vi "readMatFile.vi"(7 "Path":path, 8 "error in (no error)":errorcluster, 9 "Skip Col Idx":i32[](array[numeric]), 10 "Skip Row Idx":i32[](array[numeric]), 11 "MatOper in":refnum<class "MatOper.lvclass">) -> (0 "error out":errorcluster, 2 "Matrix":dbl[][](array[numeric]), 3 "MatOper out":refnum<class "MatOper.lvclass">)   [LabVIEW 2016, in "MatOper.lvclass"]
doc: "Read the 2D matrix data from file."
uses:
  MatOper.lvclass
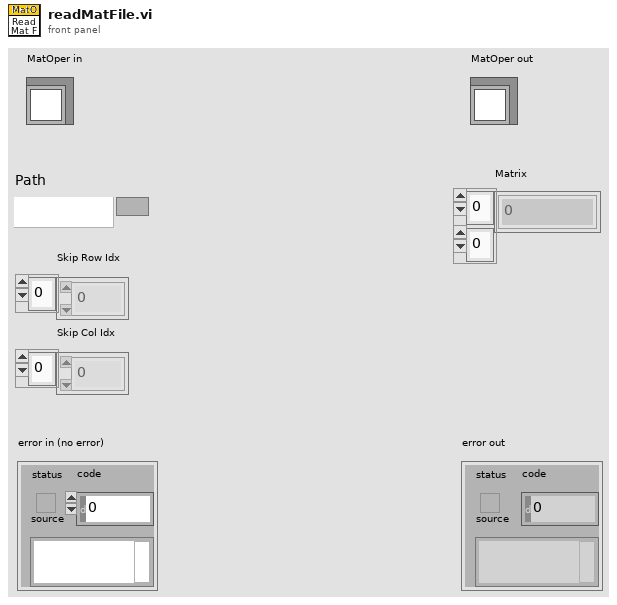
[diagram p1: front panel]
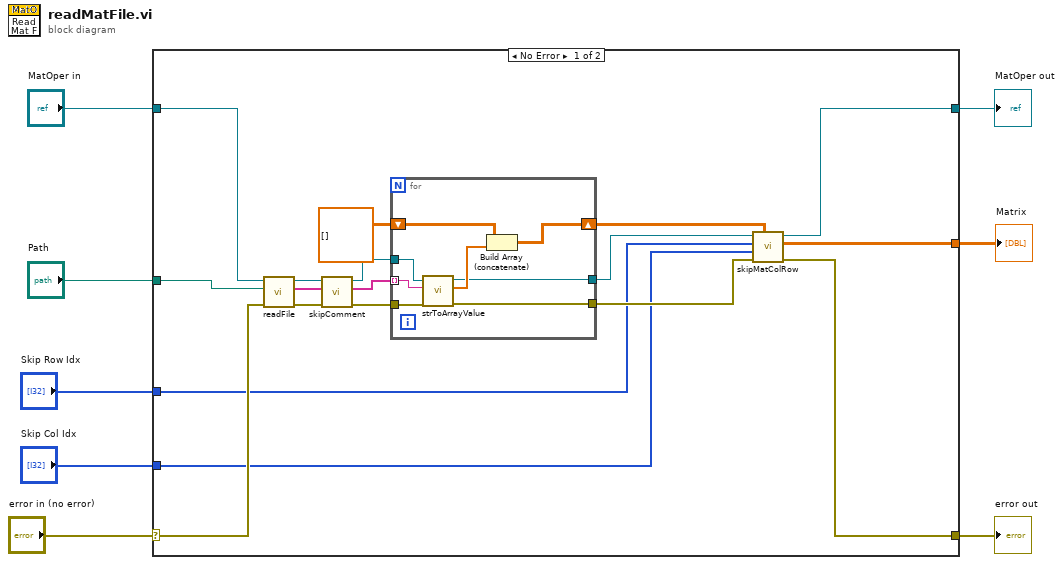
[diagram p0: block diagram]
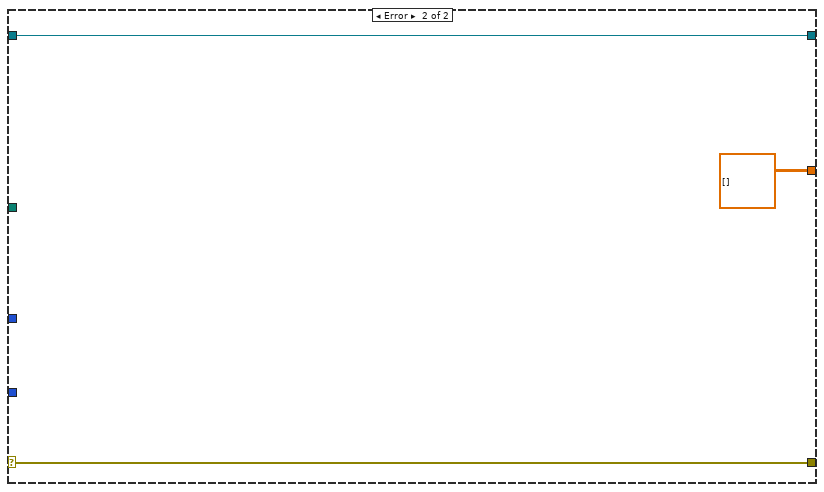
[diagram p2: hidden frame]
diagram:
  n1 = case shown="No Error" "error in (no error)" {
    selector: "error in (no error)" -> [w20 w37]
    tunnel: [w21 w37] -> w7
    tunnel: [w9 w36] -> w5
    tunnel: "MatOper in" -> [w10 w36]
    tunnel: [w22 dbl[][] [] ("Sub-Array")] -> w4
    tunnel: "Path" -> [w19 _]
    tunnel: "Skip Row Idx" -> [w18 _]
    tunnel: "Skip Col Idx" -> [w17 _]
    frame No Error {
      n2 = call "readFile.vi"("error in (no error)"=w20, "Path"=w19, "MatOper in"=w10) -> ("error out"=w15:errorcluster, "Array"=w26:string[], "MatOper out"=w13:refnum<class "MatOper.lvclass">)  [unwired: 6 in]
      n3 = call "skipComment.vi"("error in (no error)"=w15, "Content"=w26, "MatOper in"=w13) -> ("error out"=w14:errorcluster, "Modified Content"=w25:string[], "MatOper out"=w12:refnum<class "MatOper.lvclass">)  [unwired: 6 in]
      n4 = for {
        tunnel: w25 -> [w29] mode=indexing
        shift-right: [w32] -> w16
        shift-left: dbl[][] [] -> [w33]
        tunnel: w14 -> [w31]
        tunnel: [w30] -> w23
        tunnel: w12 -> [w28]
        tunnel: [w27] -> w11
        n5 = call "strToArrayValue.vi"("error in (no error)"=w31, "String"=w29, "MatOper in"=w28) -> ("error out"=w30:errorcluster, "Array"=w34:dbl[], "MatOper out"=w27:refnum<class "MatOper.lvclass">)  [unwired: 6 in]
        n6 = Build Array (concatenate)(w33, w34) -> (w32:dbl[][])
      }
      n7 = call "skipMatColRow.vi"("Matrix"=w16, "error in (no error)"=w23, "Skip Col Idx"=w17, "Skip Row Idx"=w18, "MatOper in"=w11) -> ("error out"=w21:errorcluster, "Sub-Array"=w22:dbl[][], "MatOper out"=w9:refnum<class "MatOper.lvclass">)  [unwired: 4 in]
    }
    frame Error {
    }
  }
  "error out" <- w7
  "MatOper out" <- w5
  "Matrix" <- w4
